vi "Auto Sequencer.vi"() -> ()   [LabVIEW 2019]
uses:
  <vilib>/event_ctls.llb/lveventtype.ctl
panel:
  in  "Turn \nDeceleration":bool=TRUE
  in  "Turn \nAcceleration":bool=TRUE
  in  "Unjank":bool
  in  "Sample Period (s)":dbl=0.02
  in  "Conditions":T1 {"vFinal (fps)" min=0.0; "vInitial (fps)" min=0.0}
  in  "Limits":T2={"Velocity (fps)"=6.0, "Acceleration (fps^2)"=15.0, "Jerk (fps^3)"=15.0} {"Jerk (fps^3)" min=0.0 step=5.0; "Acceleration (fps^2)" min=0.0; "Velocity (fps)" min=0.0}
  in  "Angular Accelerations":T3 {"Angular \nAccelerations" step=5.0}
  in  "Snap robot to baseline":bool
  in  "Angle Limiter":enum16{"90", "45", "15", "1"}(ring)=enum."15"
  in  "Snap to foot":bool
  in  "Center Flip":bool
  out "Saved?":bool
  in  "Time (s)":dbl(slide) scale=0.0..2.34 scale format="%#.1g"
  in  "Play":bool
  in  "Destination":u16(ring) items=["Cargo", "Rocket"]
  in  "Direction":u16(ring) items=["Left", "Right", "Other"]
  out "fps":dbl[](graph)
  in  "Append":bool
  out "WayPoints":cluster{"x":dbl, "y":dbl, "th":dbl}[](array[cluster]) {"th" format="%#_4g"}
  out "Distance (ft)":dbl format="%#.1g"
  in  "Open":i32(listbox)
  out "Path Status":bool
  out "Duration (s)":dbl format="%#.4g"
  in  "Filename":string
  in  "Save":bool
  in  "New":bool
  out "Picture":picture
  # "Trajectory Parameters"
  # "(20ms)"
  # "Interaction Options"
  # "Path Info"
  # "Directions:\nUse mouse to ...\n    move robot position (rectangle with arrow)\n    rotate robot (red arrow)\n    move waypoints (numbered circles)\nClick in open space to add a waypoint\nShift click to delete a waypoint\nHover over a waypoint and use arrow keys to nudge\n\nTime slider and Play button will run robot along path\nto test for collisions\n\nDirection and Destionation are folder selectors for files\n\nNew creates a new path at default location\n\nAppend creates a path"
  # "Interaction Options"
  # "Nicotine"
  # "1"
  # "2"
  # "3"
  # "4"
  # "5"
  # "6"
  # "7"
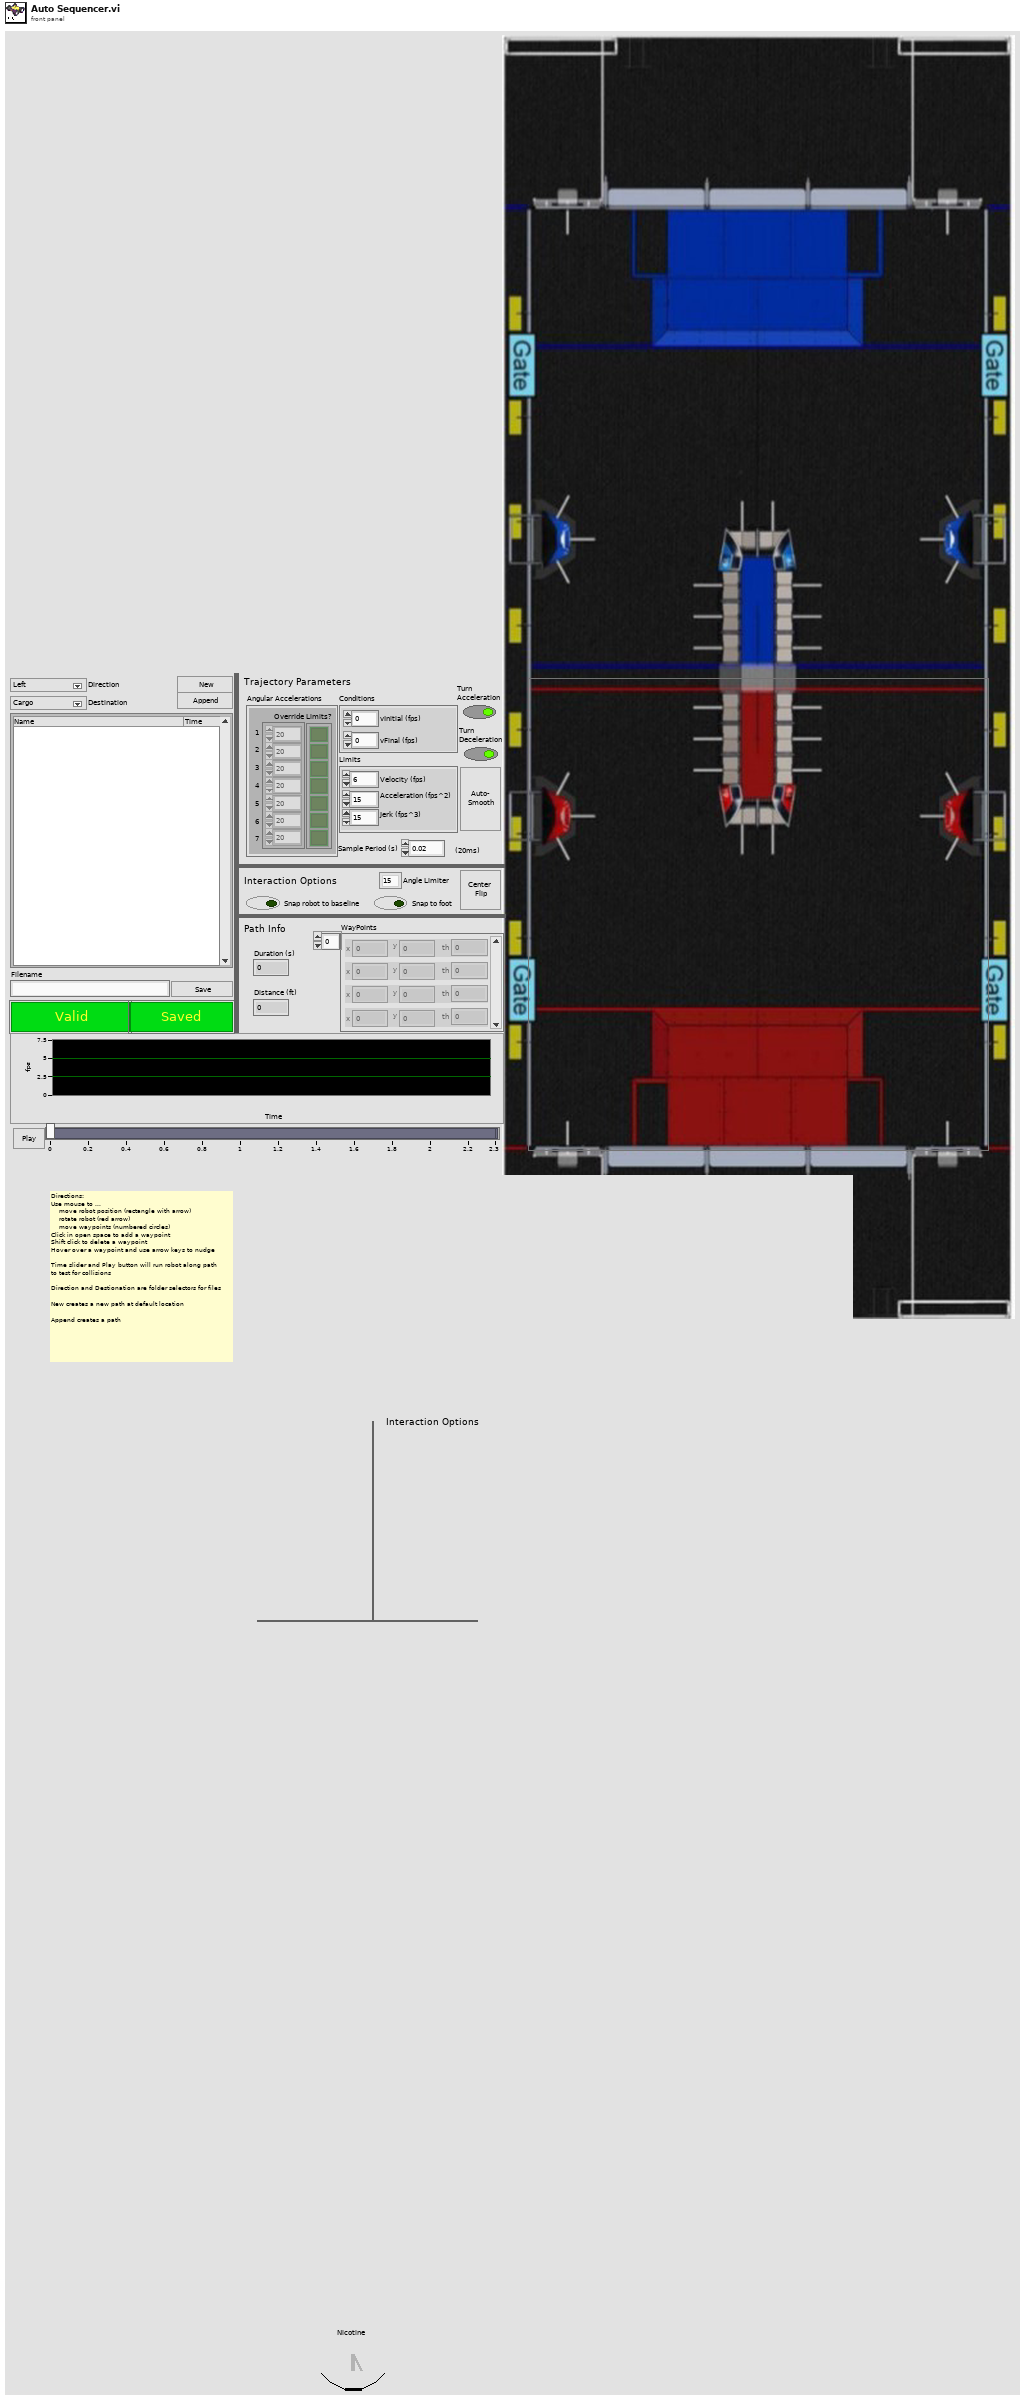
[diagram p1: front panel]
types:
  T1 = cluster{"vInitial (fps)":dbl, "vFinal (fps)":dbl}
  T2 = cluster{"Velocity (fps)":dbl, "Acceleration (fps^2)":dbl, "Jerk (fps^3)":dbl}
  T3 = cluster{"Angular \nAccelerations":dbl[], "Override Limits?":bool[]}
  T4 = cluster{"Name":string, "Color":u32, "Style":i32, "Point Style":i32, "Name Visible":bool, "Allow Drag":bool, "Annotation Mode":i32, "Plot":i32, "Index":i32, "Position":cluster{"X":dbl, "Y":dbl}, "X Scale":i32, "Y Scale":u32, "Show Arrow":bool, "Lock Name":bool, "Plot Area":i32, "Label Offset":cluster{"X":dbl, "Y":dbl}}
  T5 = cluster{"Index":i32, "Pt Test Results":enum16{"Miss", "Rect Hit", "Arrow Hit"}}
  T6 = enum16{"Accel Straight", "Const Straight", "Blend", "Circle"}
  T7 = cluster{"Velocity":dbl, "Sample Time":dbl, "Accel":dbl}
  T8 = cluster{"Segment Name":string, "Type":enum16{"Accel Straight", "Const Straight", "Blend", "Circle"}, "Traj Pos Points":cluster{"x":dbl, "y":dbl, "th":dbl}[], "Traj Vel Points":cluster{"V":dbl, "th":dbl}[], "Accel Index":i32, "Decel Index":i32}[]
  T9 = cluster{"Sample Period (s)":dbl, "Limits":cluster{"Velocity (fps)":dbl, "Acceleration (fps^2)":dbl, "Jerk (fps^3)":dbl}, "Conditions":cluster{"vInitial (fps)":dbl, "vFinal (fps)":dbl}}
  T10 = cluster{"Sample Period (s)":dbl, "Limits":cluster{"Velocity (fps)":dbl, "Acceleration (fps^2)":dbl, "Jerk (fps^3)":dbl}, "Conditions":cluster{"vInitial (fps)":dbl, "vFinal (fps)":dbl}, "Min Rads":dbl[]}
  T11 = typedef "lveventtype.ctl" = enum32{"Null", "Timeout", "Annotation Menu Selection", "Annotation Menu Selection?", "App Instance Close", "App Instance Close?", "Autoscale Range Change", "Bookmark Info Change", "Cell Edit", "Cell Edit?", "Cursor Grab", "Cursor Grab?", "Cursor Menu Selection", "Cursor Menu Selection?", "Cursor Move", "Cursor Release", "Data Change", "Direction Change", "Display State Change", "Drag Ended", "Drag Enter", "Drag Leave", "Drag Over", "Drag Source Update", "Drag Starting", "Drag Starting?", "Drop", "Exec State Change", "Key Down", "Key Down?", "Key Repeat", "Key Repeat?", "Key Up", "Listbox Double Click", "Menu Activation?", "Menu Selection (App)", "Menu Selection? (App)", "Menu Selection (User)", "Mouse Down", "Mouse Down?", "Mouse Enter", "Mouse Leave", "Mouse Move", "Mouse Up", "Mouse Wheel", "NI Security User Change (App)", "Pane Size", "Panel Close", "Panel Close?", "Panel Resize", "Plot Attribute Change", "Scale Range Change", "Shortcut Menu Activation?", "Shortcut Menu Selection (App)", "Shortcut Menu Selection? (App)", "Shortcut Menu Selection (User)", "Tree Double Click", "Tree Drag", "Tree Drag?", "Tree Drop", "Tree Drop?", "Tree Item Close", "Tree Item Close?", "Tree Item Open", "Tree Item Open?", "User Event", "Value Change"}
  T12 = typedef "LVPoint32TypeDef.ctl" = cluster{"Horizontal":i32, "Vertical":i32}
  T13 = cluster{"Shift":bool, "Ctrl":bool, "Alt":bool, "Cmd":bool, "Opt":bool}
  T14 = typedef "LVPositionTypeDef.ctl" = cluster{"Left":i32, "Top":i32}
  T15 = typedef "LVBoundsTypeDef.ctl" = cluster{"Width":u32, "Height":u32}
  T16 = cluster{"Velocity":dbl, "Accel":dbl, "Accel":dbl}
  T17 = cluster{"Sample Period (s)":dbl, "Limits":cluster{"Velocity (fps)":dbl, "Acceleration (fps^2)":dbl, "Jerk (fps^3)":dbl}, "Conditions":cluster{"vInitial (fps)":dbl, "vFinal (fps)":dbl}, "Angular Accelerations":cluster{"Angular \nAccelerations":dbl[], "Override Limits?":bool[]}}
  T18 = cluster{"Trajectory Data":cluster{"Segment Name":string, "Type":enum16{"Accel Straight", "Const Straight", "Blend", "Circle"}, "Traj Pos Points":cluster{"x":dbl, "y":dbl, "th":dbl}[], "Traj Vel Points":cluster{"V":dbl, "th":dbl}[], "Accel Index":i32, "Decel Index":i32}[], "Points":cluster{"x":dbl, "y":dbl, "th":dbl}[], cluster{"Sample Period (s)":dbl, "Limits":cluster{"Velocity (fps)":dbl, "Acceleration (fps^2)":dbl, "Jerk (fps^3)":dbl}, "Conditions":cluster{"vInitial (fps)":dbl, "vFinal (fps)":dbl}, "Angular Accelerations":cluster{"Angular \nAccelerations":dbl[], "Override Limits?":bool[]}}}
  T19 = cluster{"Snap robot to baseline":bool, "Snap to foot":bool, "Angle Limiter":enum16{"90", "45", "15", "1"}}
  T20 = cluster{i32, "Pt Test Results":enum16{"Miss", "Rect Hit", "Arrow Hit"}}
  T21 = cluster{"Trajectory Data":cluster{"Segment Name":string, "Type":enum16{"Accel Straight", "Const Straight", "Blend", "Circle"}, "Traj Pos Points":cluster{"x":dbl, "y":dbl, "th":dbl}[], "Traj Vel Points":cluster{"V":dbl, "th":dbl}[], "Accel Index":i32, "Decel Index":i32}[], "Updated Waypoints":cluster{"x":dbl, "y":dbl, "th":dbl}[], cluster{"Sample Period (s)":dbl, "Limits":cluster{"Velocity (fps)":dbl, "Acceleration (fps^2)":dbl, "Jerk (fps^3)":dbl}, "Conditions":cluster{"vInitial (fps)":dbl, "vFinal (fps)":dbl}, "Angular Accelerations":cluster{"Angular \nAccelerations":dbl[], "Override Limits?":bool[]}}}
  T22 = typedef "eventvkey.ctl" = enum16{"ASCII", "Enter", "Return", "Shift", "Ctrl", "Alt", "Cmd", "Opt", "Caps", "NumLock", "Clear", "Break", "Up", "Down", "Left", "Right", "Insert", "Delete", "Home", "End", "PageUp", "PageDown", "Escape", "Help", "Pause", "ScrollLock", "F1", "F2", "F3", "F4", "F5", "F6", "F7", "F8", "F9", "F10", "F11", "F12", "F13", "F14", "F15", "F16", "F17", "F18", "F19", "F20", "F21", "F22", "F23", "F24", "Play", "VolumeUp", "VolumeDown", "Mute", "Two Byte Char"}
  T23 = cluster{"Horizontal":dbl, "Vertical":dbl, "th":dbl}
  T24 = cluster{"Name":string, "Color":u32, "Style":i32, "Point Style":i32, "Name Visible":bool, "Allow Drag":bool, "Annotation Mode":i32, "Plot":i32, "Index":i32, "Position":cluster{"X":dbl, "Y":dbl}, "X Scale":i32, "Y Scale":u32, "Show Arrow":bool, "Lock Name":bool, "Plot Area":i32, "Label Offset":cluster{"X":dbl, "Y":dbl}}[]
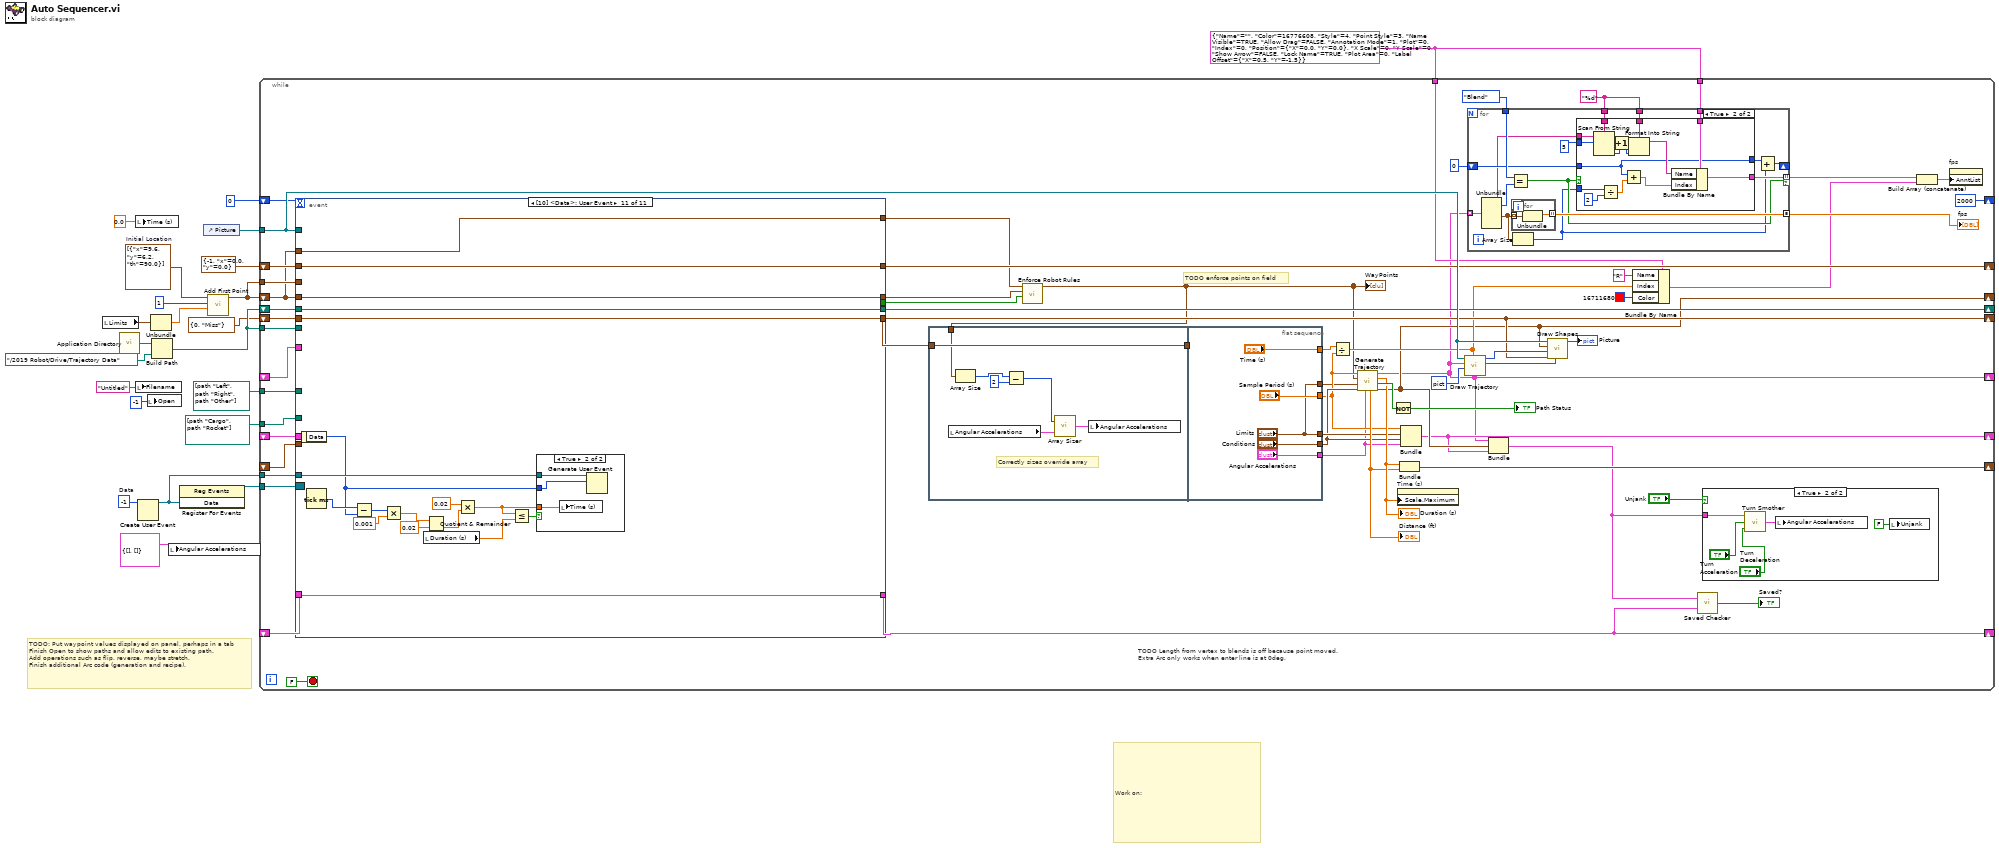
[diagram p0: block diagram]
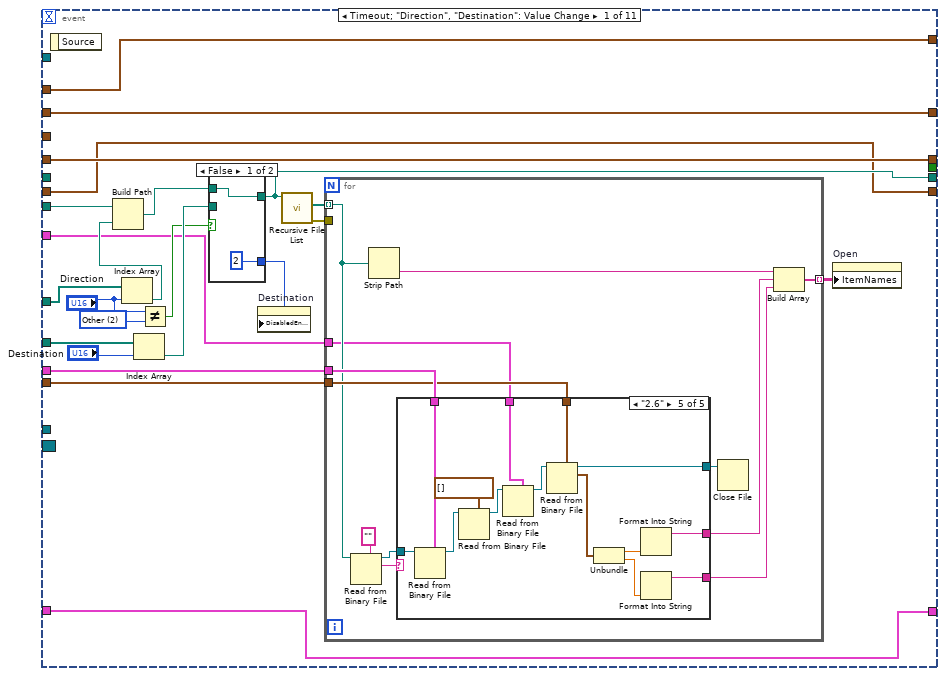
[diagram p3: hidden frame]
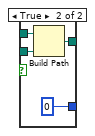
[diagram p4: hidden frame]
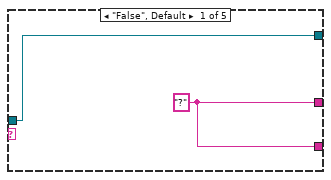
[diagram p5: hidden frame]
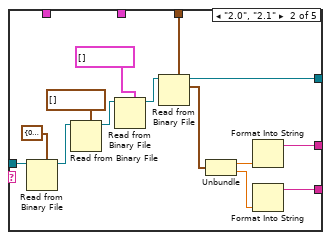
[diagram p6: hidden frame]
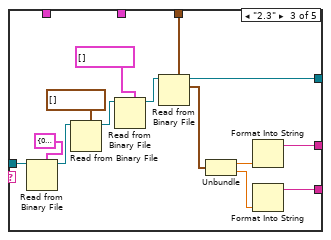
[diagram p7: hidden frame]
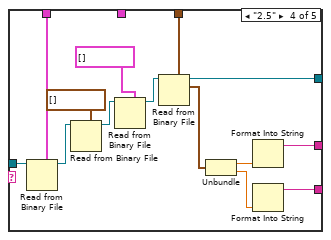
[diagram p8: hidden frame]
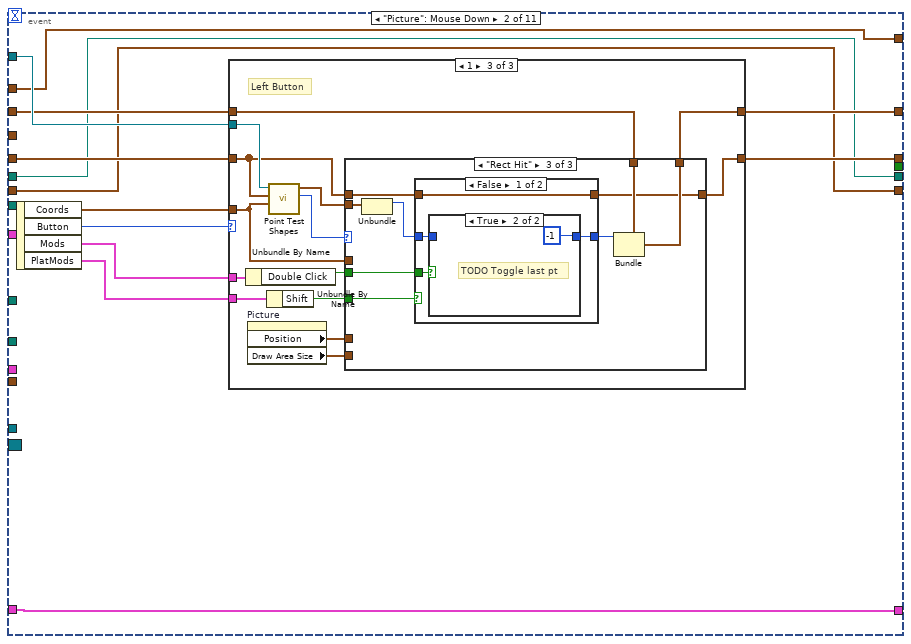
[diagram p9: hidden frame]
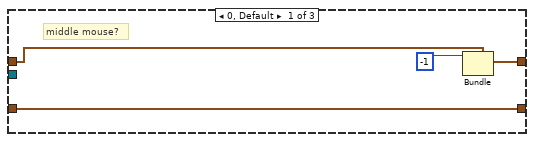
[diagram p10: hidden frame]
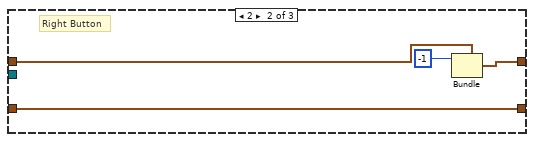
[diagram p11: hidden frame]
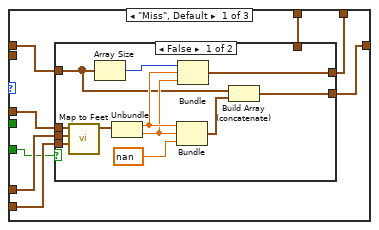
[diagram p12: hidden frame]
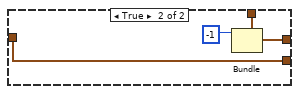
[diagram p13: hidden frame]
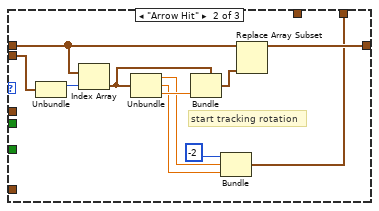
[diagram p14: hidden frame]
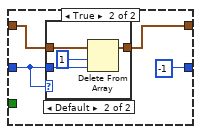
[diagram p16: hidden frame]
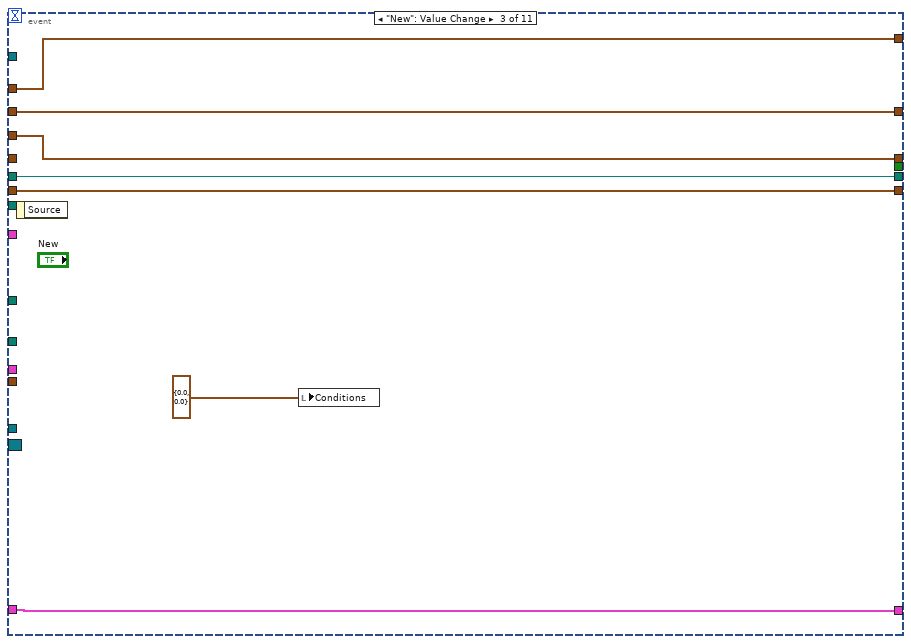
[diagram p18: hidden frame]
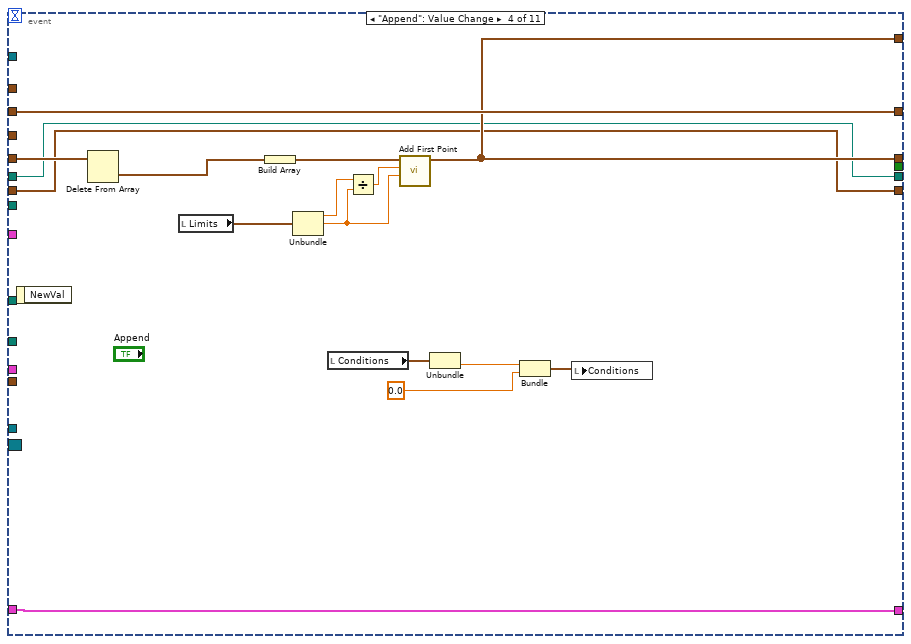
[diagram p19: hidden frame]
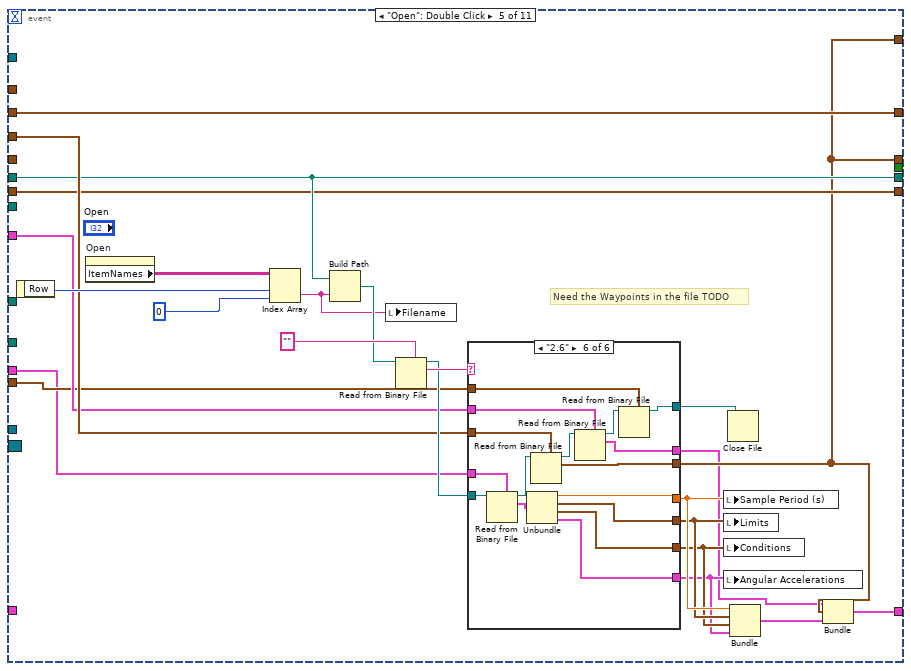
[diagram p20: hidden frame]
diagram:
  w2 = -1  # Data
  w5 = T4 {"Name"="", "Color"=16776608, "Style"=4, "Point Style"=3, "Name Visible"=TRUE, "Allow Drag"=FALSE, "Annotation Mode"=1, "Plot"=0, "Index"=0, "Position"={"X"=0.0, "Y"=0.0}, "X Scale"=0, "Y Scale"=0, "Show Arrow"=FALSE, "Lock Name"=TRUE, "Plot Area"=0, "Label Offset"={"X"=0.5, "Y"=-1.5}}
  w19 = cluster{"x":dbl, "y":dbl, "th":dbl}[] [{"x"=9.6, "y"=6.2, "th"=90.0}]  # Initial Location
  # "Work on:"
  # "TODO: Put waypoint values displayed on panel, perhaps in a tab\nFinish Open to show paths and allow edits to existing path.\nAdd operations such as flip, reverse, maybe stretch.\nFinish additional Arc code (generation and recipe)."
  n1 = local read "Limits"() -> (w13:T2)
  n2 = call <vilib>:"Application Directory.vi"() -> ("Application Directory"=w16:path)
  n3 = local write "Filename"("Untitled" ("Filename")) -> ()
  n4 = local write "Time (s)"(0.0 ("Time")) -> ()
  n5 = Create User Event(user event datatype=w2) -> (user event=w3:refnum<user-event>)  [unwired: 1 in, 1 out]
  n6 = local write "Open"(-1) -> ()
  n7 = Unbundle(w13) -> ("Acceleration (fps^2)"=w12:dbl)  [unwired: 2 out]
  n8 = Build Path(base path=w16, name or relative path=path "../2019 Robot/Drive/Trajectory Data") -> (appended path=w9:path)
  n9 = local write "Angular Accelerations"(T3 {"Angular \nAccelerations"=[], "Override Limits?"=[]} ("Angular Accelerations")) -> ()
  n10 = register-events(w3) -> (reference out=w4:refnum<event-registration>)  [unwired: 2 in, 1 out]
  n11 = control-ref of="Picture"() -> (w22:refnum<vi>)
  n12 = call "Add First Point.vi"("Accel (f/s^2)"=w12, "Time (s)"=1 ("th"), "Initial Points"=w19) -> ("Points"=w18:cluster{"x":dbl, "y":dbl, "th":dbl}[])  [unwired: 8 in]
  n13 = while {
    shift-right: [w29] -> _
    shift-left: w18 -> [w68]
    tunnel: w18 -> [w81]
    tunnel: w22 -> [w79]
    shift-right: [w62] -> _
    shift-left: cluster{i32, "x":dbl, "y":dbl} {-1, "x"=0.0, "y"=0.0} ("output cluster") -> [w80]
    shift-right: [w25] -> _
    shift-left: _ -> [w71]
    shift-right: [2000] -> _
    shift-left: 0 -> [w70]
    shift-right: [w28] -> _
    shift-left: _ -> [w67]
    shift-right: [w64] -> _
    shift-left: _ -> [w63]
    tunnel: path[] [path "Left", path "Right", path "Other"] -> [w53]
    tunnel: path[] [path "Cargo", path "Rocket"] -> [w52]
    shift-right: [w50] -> _
    shift-left: w9 -> [w51]
    tunnel: w9 -> [w49]
    shift-right: [w48] -> _
    shift-left: T5 {"Index"=0, "Pt Test Results"=enum."Miss"} ("Results") -> [w47]
    tunnel: w5 -> [w44]
    tunnel: w5 -> [w40]
    tunnel: w4 -> [w35]
    tunnel: w3 -> [w34]
    shift-right: [w27] -> _
    shift-left: _ -> [w30]
    stop <- FALSE stop-if-true
    w43 = "%d" ("Name")
    # "TODO Length from vertex to blends is off because point moved.\nExtra Arc only works when enter line is at 0deg."
    # "TODO enforce points on field"
    n14 = event shown="[10] <Data>: User Event" {
      selector: w35 -> [_ _ _ _ _ _ _ _ _ _ _]
      dyn-events: _ -> [_ _ _ _ _ _ _ _ _ _ _]
      timeout: w70 -> [_ _ _ _ _ _ _ _ _ _ _]
      tunnel: w68 -> [w122 w208 _ w314 _ w440 w477 w495 w517 w554 w571]
      tunnel: [w122 w207 w299 w312 w318 w441 w477 w496 w525 w554 w571] -> w61
      tunnel: w81 -> [_ _ w299 _ w332 _ _ _ _ _ _]
      tunnel: w79 -> [_ w206 _ _ _ w443 _ _ w523 _ _]
      tunnel: [w102 w200 w294 w301 w325 w442 w475 w489 w524 w550 w569] -> w48
      tunnel: w80 -> [w121 w205 w298 w315 w339 w437 w487 w497 w526 w553 w568]
      tunnel: [w121 w204 w298 w315 w339 w439 w487 w497 w526 w553 w568] -> w62
      tunnel: w71 -> [w100 _ _ _ w331 _ w471 _ _ _ _]
      tunnel: w51 -> [_ w201 w295 w302 w326 w431 w476 w490 w528 w552 w570]
      tunnel: [w118 w202 w297 w312 w318 w435 w473 w495 w527 w551 w572] -> w60
      tunnel: w68 -> [w118 w202 w297 _ _ w435 w473 _ w527 w551 w572]
      tunnel: w67 -> [w117 _ _ _ w324 _ w472 _ _ _ _]
      tunnel: w63 -> [w116 _ _ _ w329 _ w482 _ _ _ _]
      tunnel: [_ _ _ _ _ _ _ TRUE ("Flip Over Center") _ _ _] -> w59
      tunnel: w53 -> [w114 _ _ _ _ _ _ _ _ _ _]
      tunnel: w52 -> [w113 _ _ _ _ _ _ _ _ _ _]
      tunnel: [w109 w201 w295 w302 w326 w431 w476 w490 w528 w552 w570] -> w50
      tunnel: w49 -> [w106 _ _ _ _ _ _ _ _ _ _]
      tunnel: w47 -> [w102 w200 w294 w301 w325 _ w475 w489 w524 w550 w569]
      tunnel: w34 -> [_ _ _ _ _ _ _ _ _ w549 w567]
      tunnel: [w101 w199 w293 w300 w317 w430 w474 w488 w509 w548 w564] -> w27
      tunnel: w30 -> [w101 w199 w293 w300 _ w430 _ w488 w509 w548 w564]
      event Timeout; "Direction", "Destination": Value Change {
        w107 = u16 2 items=["Left", "Right", "Other"] ("Direction")
        n15 = event-data() -> ()  [unwired: 1 in, 1 out]
        n16 = Index Array(array=w114, index="Direction") -> (element=w110:path)
        n17 = Build Path(base path=w106, name or relative path=w110) -> (appended path=w111:path)
        n18 = Index Array(array=w113, index="Destination") -> (element=w105:path)
        n19 = Not Equal?(x="Direction", y=w107) -> (x != y?=w104:bool)
        n20 = case shown="False" w104 {
          tunnel: w111 -> [w124 w128]
          tunnel: [w124 w127] -> w109
          tunnel: w105 -> [_ w126]
          tunnel: [2 0] -> w103
          frame False {
          }
          frame True {
            n21 = Build Path(base path=w128, name or relative path=w126) -> (appended path=w127:path)
          }
        }
        n22 = property on="Destination" class="Ring (strict)"("DisabledEnum"=w103) -> ()  [unwired: 2 in, 2 out]
        n23 = call <vilib>:"Recursive File List.vi"("Folder Path"=w109) -> ("error out"=w115:errorcluster, "All Files in Dir"=w120:path[])  [unwired: 6 in, 3 out]
        n24 = for {
          tunnel: w120 -> [w130] mode=indexing
          tunnel: [w140] -> w119 mode=indexing
          tunnel: w117 -> [w135]
          tunnel: w116 -> [w134]
          tunnel: w115 -> [_]
          tunnel: w100 -> [w129]
          n25 = Read from Binary File(5:"", 11:w130) -> (2:w138:string, 3:w137:refnum<file>)  [unwired: 4 in, 2 out]
          n26 = Strip Path(path=w130) -> (name=w131:string)  [unwired: 1 out]
          n27 = case shown="\"2.6\"" w138 {
            tunnel: [w142 w156 w170 w184 w198] -> w133
            tunnel: [w142 w155 w169 w183 w197] -> w132
            tunnel: w137 -> [w141 w154 w168 w182 w196]
            tunnel: [w141 w150 w164 w178 w192] -> w136
            tunnel: w135 -> [_ _ _ w171 w186]
            tunnel: w134 -> [_ w149 w163 w177 w191]
            tunnel: w129 -> [_ _ _ _ w185]
            frame "False", Default {
              w142 = "?"
            }
            frame "2.0", "2.1" {
              n28 = Read from Binary File(5:T7 {"Velocity"=0.0, "Sample Time"=0.0, "Accel"=0.0}, 11:w154) -> (3:w153:refnum<file>)  [unwired: 4 in, 3 out]
              n29 = Read from Binary File(5:cluster{"x":dbl, "y":dbl, "th":dbl}[] [] ("Points"), 11:w153) -> (3:w152:refnum<file>)  [unwired: 4 in, 3 out]
              n30 = Read from Binary File(5:T8 [] ("Trajectory Data"), 11:w152) -> (3:w151:refnum<file>)  [unwired: 4 in, 3 out]
              n31 = Read from Binary File(5:w149, 11:w151) -> (2:w144:cluster{"Time (s)":dbl, "Distance (ft)":dbl}, 3:w150:refnum<file>)  [unwired: 4 in, 2 out]
              n32 = Unbundle(w144) -> ("Time (s)"=w148:dbl, "Distance (ft)"=w147:dbl)
              n33 = Format Into String(w148) -> (resulting string=w156:string)  [unwired: 3 in, 1 out]
              n34 = Format Into String(w147) -> (resulting string=w155:string)  [unwired: 3 in, 1 out]
            }
            frame "2.3" {
              n35 = Read from Binary File(5:T9 {"Sample Period (s)"=0.0, "Limits"={"Velocity (fps)"=0.0, "Acceleration (fps^2)"=0.0, "Jerk (fps^3)"=0.0}, "Conditions"={"vInitial (fps)"=0.0, "vFinal (fps)"=0.0}}, 11:w168) -> (3:w167:refnum<file>)  [unwired: 4 in, 3 out]
              n36 = Read from Binary File(5:cluster{"x":dbl, "y":dbl, "th":dbl}[] [] ("Points"), 11:w167) -> (3:w166:refnum<file>)  [unwired: 4 in, 3 out]
              n37 = Read from Binary File(5:T8 [] ("Trajectory Data"), 11:w166) -> (3:w165:refnum<file>)  [unwired: 4 in, 3 out]
              n38 = Read from Binary File(5:w163, 11:w165) -> (2:w158:cluster{"Time (s)":dbl, "Distance (ft)":dbl}, 3:w164:refnum<file>)  [unwired: 4 in, 2 out]
              n39 = Unbundle(w158) -> ("Time (s)"=w162:dbl, "Distance (ft)"=w161:dbl)
              n40 = Format Into String(w162) -> (resulting string=w170:string)  [unwired: 3 in, 1 out]
              n41 = Format Into String(w161) -> (resulting string=w169:string)  [unwired: 3 in, 1 out]
            }
            frame "2.5" {
              n42 = Read from Binary File(5:w171, 11:w182) -> (3:w181:refnum<file>)  [unwired: 4 in, 3 out]
              n43 = Read from Binary File(5:cluster{"x":dbl, "y":dbl, "th":dbl}[] [] ("Points"), 11:w181) -> (3:w180:refnum<file>)  [unwired: 4 in, 3 out]
              n44 = Read from Binary File(5:T8 [] ("Trajectory Data"), 11:w180) -> (3:w179:refnum<file>)  [unwired: 4 in, 3 out]
              n45 = Read from Binary File(5:w177, 11:w179) -> (2:w172:cluster{"Time (s)":dbl, "Distance (ft)":dbl}, 3:w178:refnum<file>)  [unwired: 4 in, 2 out]
              n46 = Unbundle(w172) -> ("Time (s)"=w176:dbl, "Distance (ft)"=w175:dbl)
              n47 = Format Into String(w176) -> (resulting string=w184:string)  [unwired: 3 in, 1 out]
              n48 = Format Into String(w175) -> (resulting string=w183:string)  [unwired: 3 in, 1 out]
            }
            frame "2.6" {
              n49 = Read from Binary File(5:w186, 11:w196) -> (3:w195:refnum<file>)  [unwired: 4 in, 3 out]
              n50 = Read from Binary File(5:cluster{"x":dbl, "y":dbl, "th":dbl}[] [] ("Points"), 11:w195) -> (3:w194:refnum<file>)  [unwired: 4 in, 3 out]
              n51 = Read from Binary File(5:w185, 11:w194) -> (3:w193:refnum<file>)  [unwired: 4 in, 3 out]
              n52 = Read from Binary File(5:w191, 11:w193) -> (2:w187:cluster{"Time (s)":dbl, "Distance (ft)":dbl}, 3:w192:refnum<file>)  [unwired: 4 in, 2 out]
              n53 = Unbundle(w187) -> ("Time (s)"=w190:dbl, "Distance (ft)"=w189:dbl)
              n54 = Format Into String(w190) -> (resulting string=w198:string)  [unwired: 3 in, 1 out]
              n55 = Format Into String(w189) -> (resulting string=w197:string)  [unwired: 3 in, 1 out]
            }
          }
          n56 = Close File(refnum=w136) -> ()  [unwired: 1 in, 2 out]
          n57 = Build Array(w131, w133, w132) -> (w140:string[])
        }
        n58 = property on="Open" class="MCListbox (strict)"("ItemNames"=w119) -> ()  [unwired: 2 in, 2 out]
      }
      event "Picture": Mouse Down {
        n59 = event-data() -> ("Coords"=w209:T12, "Button"=w211:u16, "Mods"=w210:cluster{"Double Click":bool, "Menu Key":bool}, "PlatMods"=w203:T13)  [unwired: 1 in]
        n60 = case shown="1" w211 {
          tunnel: w210 -> [_ _ w223]
          tunnel: w209 -> [_ _ w228]
          tunnel: w208 -> [w215 w219 w229]
          tunnel: [w215 w219 w233] -> w207
          tunnel: w206 -> [_ _ w230]
          tunnel: w205 -> [w213 w216 w224]
          tunnel: [w212 w218 w225] -> w204
          tunnel: w203 -> [_ _ w221]
          frame 0, Default {
            # "middle mouse?"
            n61 = Bundle(cluster=w213, -1) -> (w212:cluster{i32, "x":dbl, "y":dbl})  [unwired: 2 in]
          }
          frame 2 {
            # "Right Button"
            n62 = Bundle(cluster=w216, -1) -> (w218:cluster{i32, "x":dbl, "y":dbl})  [unwired: 2 in]
          }
          frame 1 {
            # "Left Button"
            n63 = Unbundle By Name(w223) -> ("Double Click"=w222:bool)
            n64 = property on="Picture" class="Pict"() -> ("Position"=w232:T14, "Draw Area Size"=w231:T15)  [unwired: 2 in, 2 out]
            n65 = Unbundle By Name(w221) -> ("Shift"=w220:bool)
            n66 = call "Point Test Shapes.vi"("Coords"=w228, "Points"=w229, "Picture in"=w230) -> ("Pt Test Results"=w227:enum16{"Miss", "Rect Hit", "Arrow Hit"}, "Results"=w226:T5)  [unwired: 7 in]
            n67 = case shown="\"Rect Hit\"" w227 {
              tunnel: w222 -> [_ _ w276]
              tunnel: w229 -> [w237 w265 w270]
              tunnel: w226 -> [_ w263 w277]
              tunnel: [w240 w266 w269] -> w233
              tunnel: w228 -> [w241 _ _]
              tunnel: w232 -> [w239 _ _]
              tunnel: w231 -> [w238 _ _]
              tunnel: [w235 w258 w273] -> w225
              tunnel: w224 -> [w234 _ w274]
              tunnel: w220 -> [w236 _ w271]
              frame "Miss", Default {
                n68 = case shown="False" w236 {
                  tunnel: w241 -> [w253 _]
                  tunnel: [w250 w257] -> w240
                  tunnel: w239 -> [w249 _]
                  tunnel: w238 -> [w248 _]
                  tunnel: w237 -> [w244 w257]
                  tunnel: [w243 w256] -> w235
                  tunnel: w234 -> [_ w254]
                  frame False {
                    n69 = call "Map to Feet.vi"("Draw Area Size"=w248, "Position"=w249, "Coords (px)"=w253) -> ("Point (ft)"=w247:cluster{dbl, dbl})  [unwired: 8 in]
                    n70 = Array Size(array=w244) -> (size(s)=w242:i32)
                    n71 = Unbundle(w247) -> (w246:dbl, w245:dbl)
                    n72 = Bundle(w246, w245, nan) -> (w251:cluster{dbl, dbl, dbl})  [unwired: 1 in]
                    n73 = Bundle(w242, w246, w245) -> (w243:cluster{i32, dbl, dbl})  [unwired: 1 in]
                    n74 = Build Array (concatenate)(w244, w251) -> (w250:cluster{"x":dbl, "y":dbl, "th":dbl}[])
                  }
                  frame True {
                    n75 = Bundle(cluster=w254, -1) -> (w256:cluster{i32, "x":dbl, "y":dbl})  [unwired: 2 in]
                  }
                }
              }
              frame "Arrow Hit" {
                # "start tracking rotation"
                n76 = Unbundle(w263) -> ("Index"=w262:i32)  [unwired: 1 out]
                n77 = Index Array(array=w265, index=w262) -> (element=w264:cluster{"x":dbl, "y":dbl, "th":dbl})
                n78 = Unbundle(w264) -> ("x"=w261:dbl, "y"=w260:dbl, "th"=w268:dbl)
                n79 = Bundle(cluster=w264, "th"=w268) -> (w267:cluster{"x":dbl, "y":dbl, "th":dbl})  [unwired: 2 in]
                n80 = Bundle(-2, "x"=w261, "y"=w260) -> (w258:cluster{i32, "x":dbl, "y":dbl})  [unwired: 1 in]
                n81 = Replace Array Subset(array=w265, new element=w267) -> (w266:cluster{"x":dbl, "y":dbl, "th":dbl}[])  [unwired: 1 in]
              }
              frame "Rect Hit" {
                n82 = Unbundle(w277) -> ("Index"=w275:i32)  [unwired: 1 out]
                n83 = case shown="False" w271 {
                  tunnel: w276 -> [w281 _]
                  tunnel: w275 -> [w280 w284]
                  tunnel: [w279 -1 ("length")] -> w272
                  tunnel: w270 -> [w278 w287]
                  tunnel: [w278 w286] -> w269
                  frame False {
                    n84 = case shown="True" w281 {
                      tunnel: w280 -> [w282 _]
                      tunnel: [w282 -1] -> w279
                      frame False {
                      }
                      frame True {
                        # "TODO Toggle last pt"
                      }
                    }
                  }
                  frame True {
                    n85 = case shown="Default" w284 {
                      tunnel: w287 -> [w288 w292]
                      tunnel: w284 -> [_ w291]
                      tunnel: [w288 w289] -> w286
                      frame 0 {
                      }
                      frame Default {
                        n86 = Delete From Array(array=w292, length=1, index=w291) -> (array with subset deleted=w289:cluster{"x":dbl, "y":dbl, "th":dbl}[])  [unwired: 1 out]
                      }
                    }
                  }
                }
                n87 = Bundle(cluster=w274, w272) -> (w273:cluster{i32, "x":dbl, "y":dbl})  [unwired: 2 in]
              }
            }
          }
        }
      }
      event "New": Value Change {
        n88 = event-data() -> ()  [unwired: 1 in, 1 out]
        n89 = local write "Conditions"(T1 {"vInitial (fps)"=0.0, "vFinal (fps)"=0.0} ("Conditions")) -> ()
      }
      event "Append": Value Change {
        n90 = event-data() -> ()  [unwired: 1 in, 1 out]
        n91 = Delete From Array(array=w314) -> (deleted portion=w311:cluster{"x":dbl, "y":dbl, "th":dbl})  [unwired: 2 in, 1 out]
        n92 = local read "Limits"() -> (w305:T2)
        n93 = Build Array(w311) -> (w310:cluster{"x":dbl, "y":dbl, "th":dbl}[])
        n94 = Unbundle(w305) -> ("Velocity (fps)"=w304:dbl, "Acceleration (fps^2)"=w303:dbl)  [unwired: 1 out]
        n95 = local read "Conditions"() -> (w309:T1)
        n96 = Divide(x=w304, y=w303) -> (x/y=w313:dbl)
        n97 = call "Add First Point.vi"("Accel (f/s^2)"=w303, "Time (s)"=w313, "Initial Points"=w310) -> ("Points"=w312:cluster{"x":dbl, "y":dbl, "th":dbl}[])  [unwired: 8 in]
        n98 = Unbundle(w309) -> ("vFinal (fps)"=w308:dbl)  [unwired: 1 out]
        n99 = Bundle("vFinal (fps)"=w308, 0.0) -> (w307:cluster{"vFinal (fps)":dbl, dbl})  [unwired: 1 in]
        n100 = local write "Conditions"(w307) -> ()
      }
      event "Open": Double Click {
        # "Need the Waypoints in the file TODO"
        n101 = event-data() -> ("Row"=w337:i32)  [unwired: 1 in]
        n102 = property on="Open" class="MCListbox (strict)"() -> ("ItemNames"=w338:string[][])  [unwired: 2 in, 2 out]
        n103 = Index Array(array=w338, index (row)=w337, index (col)=0 ("disabled index (col)")) -> (element=w327:string)
        n104 = Build Path(base path=w326, name or relative path=w327) -> (appended path=w328:path)
        n105 = local write "Filename"(w327) -> ()
        n106 = Read from Binary File(5:"", 11:w328) -> (2:w334:string, 3:w333:refnum<file>)  [unwired: 4 in, 2 out]
        n107 = case shown="\"2.6\"" w334 {
          tunnel: w333 -> [w342 w359 w375 w391 w411 w428]
          tunnel: w324 -> [_ _ _ _ _ w417]
          tunnel: w332 -> [_ w357 w373 w389 w409 w426]
          tunnel: [_ w356 w372 w388 w408 w425] -> w318
          tunnel: w331 -> [_ w355 w371 w387 w407 w424]
          tunnel: w329 -> [_ w353 w369 w385 w405 w422]
          tunnel: [w342 w351 w367 w383 w403 w420] -> w330
          tunnel: [_ w349 w366 w382 w402 w419] -> w323
          tunnel: [_ w348 w365 w381 w401 w418] -> w322
          tunnel: [_ _ w364 w380 w400 w416] -> w321
          tunnel: [T3 {"Angular \nAccelerations"=[], "Override Limits?"=[]} ("Angular Accelerations") T3 {"Angular \nAccelerations"=[], "Override Limits?"=[]} ("Angular Accelerations") T3 {"Angular \nAccelerations"=[], "Override Limits?"=[]} ("Angular Accelerations") T3 {"Angular \nAccelerations"=[], "Override Limits?"=[]} ("Angular Accelerations") w394 w415] -> w320
          tunnel: [T8 [] ("Trajectory Data") w343 w361 w377 w393 w414] -> w316
          frame "False", Default {
          }
          frame "2.0", "2.1" {
            n108 = Read from Binary File(5:T7 {"Velocity"=0.0, "Sample Time"=0.0, "Accel"=0.0}, 11:w359) -> (2:w360:T7, 3:w358:refnum<file>)  [unwired: 4 in, 2 out]
            n109 = Read from Binary File(5:w357, 11:w358) -> (2:w356:cluster{"x":dbl, "y":dbl, "th":dbl}[], 3:w354:refnum<file>)  [unwired: 4 in, 2 out]
            n110 = Unbundle(w360) -> ("Velocity"=w347:dbl, "Sample Time"=w349:dbl, "Accel"=w346:dbl)
            n111 = Read from Binary File(5:w355, 11:w354) -> (2:w343:T8, 3:w352:refnum<file>)  [unwired: 4 in, 2 out]
            n112 = Read from Binary File(5:w353, 11:w352) -> (3:w351:refnum<file>)  [unwired: 4 in, 3 out]
            n113 = Bundle("Velocity"=w347, "Accel"=w346, "Accel"=1000.0) -> (w348:T16)  [unwired: 1 in]
          }
          frame "2.3" {
            n114 = Read from Binary File(5:T9 {"Sample Period (s)"=0.0, "Limits"={"Velocity (fps)"=0.0, "Acceleration (fps^2)"=0.0, "Jerk (fps^3)"=0.0}, "Conditions"={"vInitial (fps)"=0.0, "vFinal (fps)"=0.0}}, 11:w375) -> (2:w376:T9, 3:w374:refnum<file>)  [unwired: 4 in, 2 out]
            n115 = Unbundle(w376) -> ("Sample Period (s)"=w366:dbl, "Limits"=w365:T2, "Conditions"=w364:T1)
            n116 = Read from Binary File(5:w373, 11:w374) -> (2:w372:cluster{"x":dbl, "y":dbl, "th":dbl}[], 3:w370:refnum<file>)  [unwired: 4 in, 2 out]
            n117 = Read from Binary File(5:w371, 11:w370) -> (2:w361:T8, 3:w368:refnum<file>)  [unwired: 4 in, 2 out]
            n118 = Read from Binary File(5:w369, 11:w368) -> (3:w367:refnum<file>)  [unwired: 4 in, 3 out]
          }
          frame "2.4" {
            n119 = Read from Binary File(5:T9 {"Sample Period (s)"=0.0, "Limits"={"Velocity (fps)"=0.0, "Acceleration (fps^2)"=0.0, "Jerk (fps^3)"=0.0}, "Conditions"={"vInitial (fps)"=0.0, "vFinal (fps)"=0.0}}, 11:w391) -> (2:w392:T9, 3:w390:refnum<file>)  [unwired: 4 in, 2 out]
            n120 = Unbundle(w392) -> ("Sample Period (s)"=w382:dbl, "Limits"=w381:T2, "Conditions"=w380:T1)
            n121 = Read from Binary File(5:w389, 11:w390) -> (2:w388:cluster{"x":dbl, "y":dbl, "th":dbl}[], 3:w386:refnum<file>)  [unwired: 4 in, 2 out]
            n122 = Read from Binary File(5:w387, 11:w386) -> (2:w377:T8, 3:w384:refnum<file>)  [unwired: 4 in, 2 out]
            n123 = Read from Binary File(5:w385, 11:w384) -> (3:w383:refnum<file>)  [unwired: 4 in, 3 out]
          }
          frame "2.5" {
            n124 = Read from Binary File(5:T10 {"Sample Period (s)"=0.0, "Limits"={"Velocity (fps)"=0.0, "Acceleration (fps^2)"=0.0, "Jerk (fps^3)"=0.0}, "Conditions"={"vInitial (fps)"=0.0, "vFinal (fps)"=0.0}, "Min Rads"=[20.0, 20.0, 20.0, 20.0, 20.0]}, 11:w411) -> (2:w412:T10, 3:w410:refnum<file>)  [unwired: 4 in, 2 out]
            n125 = Unbundle(w412) -> ("Sample Period (s)"=w402:dbl, "Limits"=w401:T2, "Conditions"=w400:T1, "Min Rads"=w396:dbl[])
            n126 = Array Size(array=w396) -> (size(s)=w397:i32)
            n127 = for {
              N: w397 -> [_]
              tunnel: [TRUE] -> w395 mode=indexing
            }
            n128 = Read from Binary File(5:w409, 11:w410) -> (2:w408:cluster{"x":dbl, "y":dbl, "th":dbl}[], 3:w406:refnum<file>)  [unwired: 4 in, 2 out]
            n129 = Read from Binary File(5:w407, 11:w406) -> (2:w393:T8, 3:w404:refnum<file>)  [unwired: 4 in, 2 out]
            n130 = Bundle(cluster=T3 {"Angular \nAccelerations"=[], "Override Limits?"=[]} ("Angular Accelerations"), "Angular \nAccelerations"=w396, "Override Limits?"=w395) -> (w394:T3)
            n131 = Read from Binary File(5:w405, 11:w404) -> (3:w403:refnum<file>)  [unwired: 4 in, 3 out]
          }
          frame "2.6" {
            n132 = Read from Binary File(5:w417, 11:w428) -> (2:w429:T17, 3:w427:refnum<file>)  [unwired: 4 in, 2 out]
            n133 = Unbundle(w429) -> ("Sample Period (s)"=w419:dbl, "Limits"=w418:T2, "Conditions"=w416:T1, "Angular Accelerations"=w415:T3)
            n134 = Read from Binary File(5:w426, 11:w427) -> (2:w425:cluster{"x":dbl, "y":dbl, "th":dbl}[], 3:w423:refnum<file>)  [unwired: 4 in, 2 out]
            n135 = Read from Binary File(5:w424, 11:w423) -> (2:w414:T8, 3:w421:refnum<file>)  [unwired: 4 in, 2 out]
            n136 = Read from Binary File(5:w422, 11:w421) -> (3:w420:refnum<file>)  [unwired: 4 in, 3 out]
          }
        }
        n137 = local write "Sample Period (s)"(w323) -> ()
        n138 = local write "Limits"(w322) -> ()
        n139 = local write "Conditions"(w321) -> ()
        n140 = local write "Angular Accelerations"(w320) -> ()
        n141 = Close File(refnum=w330) -> ()  [unwired: 1 in, 2 out]
        n142 = Bundle("Sample Period (s)"=w323, "Limits"=w322, "Conditions"=w321, "Angular Accelerations"=w320) -> (w319:T17)  [unwired: 1 in]
        n143 = Bundle("Trajectory Data"=w316, "Points"=w318, w319) -> (w317:T18)  [unwired: 1 in]
      }
      event "Picture": Mouse Move; "Picture": Mouse Up {
        n144 = event-data() -> ("Type"=w438:T11, "Coords"=w444:T12)  [unwired: 1 in]
        n145 = Unbundle(w437) -> (w436:i32)  [unwired: 2 out]
        n146 = case shown="-1" w436 {
          selector: w436 -> [w454 _]
          tunnel: w444 -> [w463 w470]
          tunnel: w443 -> [w449 w469]
          tunnel: [w461 w468] -> w442
          tunnel: [w458 w467] -> w441
          tunnel: w440 -> [w459 w467]
          tunnel: [w455 w466] -> w439
          tunnel: w437 -> [w445 w466]
          tunnel: w438 -> [w456 _]
          tunnel: "Snap to foot" -> [w451 _]
          tunnel: "Snap robot to baseline" -> [w452 _]
          tunnel: "Angle Limiter" -> [w453 _]
          frame Default {
            # "Mouse up changes indes to break tracking,\notherwise update coords"
            n147 = property on="Picture" class="Pict"() -> ("Position"=w464:T14, "Draw Area Size"=w465:T15)  [unwired: 2 in, 2 out]
            n148 = Bundle("Snap robot to baseline"=w452, "Snap to foot"=w451, "Angle Limiter"=w453) -> (w450:T19)  [unwired: 1 in]
            n149 = call "Map to Feet.vi"("Draw Area Size"=w465, "Position"=w464, "Coords (px)"=w463) -> ("Point (ft)"=w462:cluster{dbl, dbl})  [unwired: 8 in]
            n150 = Equal?(x=lveventtype."Mouse Up" ("Type"), y=w456) -> (x = y?=w448:bool)
            n151 = call "Handle Pos and Rot.vi"("Mouse Up"=w448, "Picture in"=w449, "Option"=w450, "Coord (ft)"=w462, "Index"=w454, "Points in"=w459) -> ("Points out"=w458:cluster{"x":dbl, "y":dbl, "th":dbl}[])  [unwired: 5 in]
            n152 = Bundle(cluster=w445, -1) -> (w446:cluster{i32, "x":dbl, "y":dbl})  [unwired: 2 in]
            n153 = Bundle(w454, "Pt Test Results"=enum16{"Miss", "Rect Hit", "Arrow Hit"}."Rect Hit") -> (w461:T20)  [unwired: 1 in]
            n154 = Select(t=w446, s=w448, f=w445) -> (s? t:f=w455:cluster{i32, "x":dbl, "y":dbl})
          }
          frame -1 {
            n155 = call "Point Test Shapes.vi"("Coords"=w470, "Points"=w467, "Picture in"=w469) -> ("Results"=w468:T5)  [unwired: 7 in, 1 out]
          }
        }
      }
      event "Save": Value Change {
        n156 = event-data() -> ()  [unwired: 1 in, 1 out]
        n157 = Build Path(base path=w476, name or relative path="Filename") -> (appended path=w480:path)
        n158 = Write to Binary File(file (use dialog)=w480, data="2.6") -> (refnum out=w479:refnum<file>)  [unwired: 4 in, 2 out]
        n159 = Write to Binary File(file (use dialog)=w479, data=w472) -> (refnum out=w485:refnum<file>)  [unwired: 4 in, 2 out]
        n160 = Write to Binary File(file (use dialog)=w485, data=w473) -> (refnum out=w484:refnum<file>)  [unwired: 4 in, 2 out]
        n161 = Write to Binary File(file (use dialog)=w484, data=w471) -> (refnum out=w483:refnum<file>)  [unwired: 4 in, 2 out]
        n162 = Write to Binary File(file (use dialog)=w483, data=w482) -> (refnum out=w481:refnum<file>)  [unwired: 4 in, 2 out]
        n163 = Close File(refnum=w481) -> ()  [unwired: 1 in, 2 out]
        n164 = Bundle("Trajectory Data"=w471, "Updated Waypoints"=w473, w472) -> (w474:T21)  [unwired: 1 in]
      }
      event "Time (s)", "Snap to foot", "Angle Limiter", "Snap robot to baseline", "Limits", "Sample Period (s)", "Center Flip", "Conditions": Value Change {
        # "Changes to any of these control will run the diagram to update the preview"
        n165 = event-data() -> ("CtlRef"=w493:refnum<vi>)  [unwired: 1 in]
        n166 = control-ref of="Center Flip"() -> (w494:refnum<vi>)
        n167 = Equal?(x=w494, y=w493) -> (x = y?=w492:bool)
        n168 = case shown="True" w492 {
          tunnel: w495 -> [w498 w500]
          tunnel: [w498 w499] -> w496
          frame False {
          }
          frame True {
            n169 = for {
              tunnel: w500 -> [w508] mode=indexing
              tunnel: [w501] -> w499 mode=indexing
              n170 = Unbundle(w508) -> ("x"=w507:dbl, "y"=w503:dbl, "th"=w502:dbl)
              n171 = Negate(x=w507) -> (-x=w506:dbl)
              n172 = Add(x=27.0 ("y"), y=w506) -> (x+y=w504:dbl)
              n173 = Bundle(w504, "y"=w503, "th"=w502) -> (w501:cluster{dbl, "y":dbl, "th":dbl})  [unwired: 1 in]
            }
          }
        }
      }
      event Key Down?; event type 5.0.x8000000b {
        n174 = event-data() -> ("VKey"=w513:T22)  [unwired: 1 in]
        n175 = local read "Snap robot to baseline"() -> (w522:bool)
        n176 = local read "Angle Limiter"() -> (w520:enum16{"90", "45", "15", "1"})
        n177 = local read "Snap to foot"() -> (w521:bool)
        n178 = case shown="\"Down\"" w513 {
          tunnel: [cluster{dbl, dbl} {0.0, 0.0} ("Coord (ft)") cluster{dbl, dbl} {0.0, 0.1} ("Coord (ft)") cluster{dbl, dbl} {0.0, -0.1} ("Coord (ft)") cluster{dbl, dbl} {-0.1, 0.0} ("Coord (ft)") cluster{dbl, dbl} {0.1, 0.0} ("Coord (ft)")] -> w515
          tunnel: [_ w539 w541 w543 w545] -> w511
          tunnel: TRUE ("Delta") -> [_ w539 w541 w543 w545]
          frame Default {
          }
          frame "Up" {
          }
          frame "Down" {
          }
          frame "Left" {
          }
          frame "Right" {
          }
        }
        n179 = Unbundle(w524) -> ("Index"=w518:i32, "Pt Test Results"=w512:enum16{"Miss", "Rect Hit", "Arrow Hit"})
        n180 = Bundle("Snap robot to baseline"=w522, "Snap to foot"=w521, "Angle Limiter"=w520) -> (w519:T19)  [unwired: 1 in]
        n181 = case shown="\"Miss\"" w512 {
          tunnel: [w529 w537] -> w525
          tunnel: w523 -> [_ w536]
          tunnel: w519 -> [_ w535]
          tunnel: w518 -> [_ w534]
          tunnel: w517 -> [w529 w533]
          tunnel: TRUE ("Delta") -> [_ w532]
          tunnel: w515 -> [_ w531]
          tunnel: w511 -> [_ w530]
          tunnel: [_ w530] -> w510
          frame "Miss" {
          }
          frame "Rect Hit", Default {
            n182 = call "Handle Pos and Rot.vi"("Delta"=w532, "Picture in"=w536, "Option"=w535, "Coord (ft)"=w531, "Index"=w534, "Points in"=w533) -> ("Points out"=w537:cluster{"x":dbl, "y":dbl, "th":dbl}[])  [unwired: 5 in]
          }
        }
        n183 = event-data("Discard?"=w510) -> ()  [unwired: 1 in, 1 out]
      }
      event "Play": Value Change {
        n184 = event-data() -> ()  [unwired: 1 in, 1 out]
        n185 = Tick Count (ms)() -> (millisecond timer value=w547:u32)
        n186 = Generate User Event(user event=w549, event data cluster=w547) -> ()  [unwired: 2 in, 2 out]
      }
      event User Event {
        n187 = event-data() -> ("Data"=w560:i32)  [unwired: 1 in]
        n188 = Tick Count (ms)() -> (millisecond timer value=w563:u32)
        n189 = Subtract(x=w563, y=w560) -> (x-y=w562:u32)
        n190 = Multiply(x=w562, y=0.001) -> (x*y=w559:dbl)
        n191 = local read "Duration (s)"() -> (w565:dbl)
        n192 = Quotient & Remainder(x=w559, y=0.02) -> (floor(x/y)=w557:dbl)  [unwired: 1 out]
        n193 = Multiply(x=0.02, y=w557) -> (x*y=w556:dbl)
        n194 = Less Or Equal?(x=w556, y=w565) -> (x <= y?=w566:bool)
        n195 = case shown="True" w566 {
          tunnel: w567 -> [_ w575]
          tunnel: w560 -> [_ w573]
          tunnel: w556 -> [_ w574]
          frame False {
          }
          frame True {
            n196 = local write "Time (s)"(w574) -> ()
            n197 = Generate User Event(user event=w575, event data cluster=w573) -> ()  [unwired: 2 in, 2 out]
          }
        }
      }
    }
    n198 = flat-sequence {
      tunnel: w48 -> [w94]
      tunnel: [w94] -> w32
      tunnel: w31 -> [w93]
      tunnel: ["Time (s)"] -> w76
      tunnel: ["Sample Period (s)"] -> w56
      tunnel: ["Conditions"] -> w57
      tunnel: ["Limits"] -> w58
      tunnel: ["Limits"] -> w55
      tunnel: ["Angular Accelerations"] -> w33
      tunnel: w32 -> [_]
      frame #0 {
        # "Correctly sizes override array"
        n199 = local read "Angular Accelerations"() -> (w92:T3)
        n200 = Array Size(array=w93) -> (size(s)=w90:i32)
        n201 = Subtract(x=w90, y=2) -> (x-y=w88:i32)
        n202 = call "Array Sizer.vi"("Angular Accelerations"=w92, "Numeric"=w88) -> ("output cluster"=w91:T3)
        n203 = local write "Angular Accelerations"(w91) -> ()
      }
      frame #1 {
      }
    }
    n204 = call "Enforce Robot Rules.vi"("Disable"=w59, "New Points"=w61, "Original Points"=w60) -> ("Points out"=w31:cluster{"x":dbl, "y":dbl, "th":dbl}[])  [unwired: 8 in]
    "WayPoints" <- w31
    n205 = Divide(x=w76, y=w56) -> (x/y=w42:dbl)
    n206 = call "Generate Trajectory.vi"("Overrides 2"=w33, "Conditions"=w57, "Limits"=w55, "WayPoints"=w31, "Sample Period (s)"=w56) -> ("Updated Waypoints"=w29:cluster{"x":dbl, "y":dbl, "th":dbl}[], "Valid"=w73:bool, "Time (s)"=w66:dbl, "Trajectory Data"=w25:T8, "Distance (ft)"=w65:dbl)  [unwired: 2 in]
    "Duration (s)" <- w66
    "Distance (ft)" <- w65
    n207 = Not(x=w73) -> (.not. x?=→"Path Status":bool)
    n208 = property on="Time (s)" class="Slide (strict)"("Scale.Maximum"=w66) -> ()  [unwired: 2 in, 2 out]
    n209 = Bundle("Time (s)"=w66, "Distance (ft)"=w65) -> (w64:cluster{"Time (s)":dbl, "Distance (ft)":dbl})  [unwired: 1 in]
    n210 = Bundle("Sample Period (s)"=w56, "Limits"=w58, "Conditions"=w57, "Angular Accelerations"=w33) -> (w28:T17)  [unwired: 1 in]
    n211 = call "Draw Trajectory.vi"("Robot Index"=w42, "new picture in"=picture data[5B] ("new picture"), "Trajectory Data"=w25, "Picture in"=w79) -> ("Output Point"=w75:T23, "new picture"=w77:picture)  [unwired: 5 in, 1 out]
    n212 = for {
      tunnel: w25 -> [w591] mode=indexing
      tunnel: [w590] -> w54 mode=concatenating
      tunnel: T6."Blend" ("Type") -> [w589]
      shift-right: [w578] -> _
      shift-left: 0 -> [w586]
      tunnel: [w581] -> w37 mode=indexing if=w580
      tunnel: w44 -> [w585]
      tunnel: w43 -> [w583]
      tunnel: w43 -> [w582]
      n213 = Unbundle(w591) -> ("Segment Name"=w584:string, "Type"=w588:T6, "Traj Vel Points"=w587:cluster{"V":dbl, "th":dbl}[])  [unwired: 3 out]
      n214 = Equal?(x=w589, y=w588) -> (x = y?=w580:bool)
      n215 = for {
        tunnel: w587 -> [w608] mode=indexing
        tunnel: [w607] -> w590 mode=indexing
        n216 = Unbundle(w608) -> ("V"=w607:dbl)  [unwired: 1 out]
      }
      n217 = Array Size(array=w587) -> (size(s)=w577:i32)
      n218 = case shown="True" w580 {
        tunnel: w586 -> [w592 w600]
        tunnel: [w592 w600] -> w579
        tunnel: w585 -> [_ w606]
        tunnel: w584 -> [_ w605]
        tunnel: w583 -> [_ w604]
        tunnel: w582 -> [_ w603]
        tunnel: [_ w601] -> w581
        tunnel: w577 -> [_ w597]
        tunnel: 5 -> [_ w596]
        frame False {
        }
        frame True {
          n219 = Scan From String(format string=w604, input string=w605, initial scan location=w596) -> (output 1=w594:i32)  [unwired: 2 in, 3 out]
          n220 = Divide(x=w597, y=2) -> (x/y=w598:dbl)
          n221 = Increment(x=w594) -> (x+1=w593:i32)
          n222 = Add(x=w600, y=w598) -> (x+y=w595:dbl)
          n223 = Format Into String(format string=w603, w593) -> (resulting string=w602:string)  [unwired: 2 in, 1 out]
          n224 = Bundle By Name(cluster=w606, "Name"=w602, "Index"=w595) -> (w601:T4)
        }
      }
      n225 = Add(x=w579, y=w577) -> (x+y=w578:i32)
    }
    "fps" <- w54
    n226 = Bundle("Trajectory Data"=w25, "Updated Waypoints"=w29, w28) -> (w23:T21)  [unwired: 1 in]
    n227 = call "Draw Shapes.vi"("Output Point"=w75, "Results"=w48, "new picture in"=w77, "Points"=w29, "Picture in"=w79) -> ("new picture out"=→"Picture":picture)  [unwired: 6 in]
    n228 = Bundle By Name(cluster=w40, "Name"="R", "Index"=w42, "Color"=u32 16711680) -> (w38:T4)
    n229 = call "Saved Checker.vi"("comp A"=w27, "comp B"=w23) -> ("Unsaved"=→"Saved?":bool)
    n230 = case shown="True" "Unjank" {
      tunnel: w23 -> [_ w86]
      frame False {
      }
      frame True {
        n231 = call "Turn Smother.vi"("Ignore Deceleration"="Turn \nDeceleration", "Ignore Acceleration"="Turn \nAcceleration", "output cluster"=w86) -> ("Angular Accelerations"=w85:T3)
        n232 = local write "Angular Accelerations"(w85) -> ()
        n233 = local write "Unjank"(FALSE ("Unjank")) -> ()
      }
    }
    n234 = Build Array (concatenate)(w37, w38) -> (w36:T24)
    n235 = property on="fps" class="WFGraph (strict)"("AnntList"=w36) -> ()  [unwired: 2 in, 2 out]
  }
